vi "Dashboard Main.vi"() -> ()   [LabVIEW 2012]
panel:
  out "Up to Speed":bool
  in  "Tab Control":enum32{"Home", "Debugging"}(tab)
  out "Drive Speed":dbl
  out "Angle of shooter":dbl
  out "Low":bool
  out "Medium":bool
  out "High":bool
  out "Coordinates":cluster{"Y":dbl[], "Y":dbl[]}[](graph)
  out "Speed of shooter":dbl
  out "Distance from target":dbl
  out "Mode":enum8{"Tele-Op", "Auto", "Test", ""}(ring)=enum."Test"
  out "Camera IP":string
  out "JS1 Z":dbl(slide) scale=-1.0..1.0 scale format="%#_2e"
  out "JS2 Z":dbl(slide) scale=-1.0..1.0 scale format="%#_2e"
  out "Joystick 1":cluster{"X":dbl, "Y":dbl}[](graph)
  out "Joystick 2":cluster{"X":dbl, "Y":dbl}[](graph)
  out "JS Buttons 1":T1
  out "JS Buttons 2":T1
  out "MotorSlide4":dbl(slide) scale=-1.0..1.0 scale format="%#_2e"
  out "MotorSlide3":dbl(slide) scale=-1.0..1.0 scale format="%#_2e"
  out "MotorSlide2":dbl(slide) scale=-1.0..1.0 scale format="%#_2e"
  in  "MotorName3":string="Front Left"
  in  "MotorName4":string="Front Right"
  in  "MotorName1":string="Rear Left"
  in  "MotorName2":string="Rear Right"
  out "MotorChart4":dbl(graph)
  out "MotorChart3":dbl(graph)
  out "MotorChart2":dbl(graph)
  out "MotorSlide1":dbl(slide) scale=-1.0..1.0 scale format="%#_2e"
  out "MotorChart1":dbl(graph)
  out "Battery Value":dbl(slide) scale=0.0..14.0 scale format="%#_2e"
  out "Robot IP":string
  out "Battery":sgl(graph)
  in  "Viewer":T2(tab)
  out "Image Error Message":string="Timeout in Camera Communications"
  in  "Video Enable":bool=TRUE
  out "Camera Image":T3(plugin-control)
  out "Buttons 1":cluster{"1":bool, "2":bool, "3":bool}
  out "Kinect 1":cluster{"X":dbl, "Y":dbl, "Z":dbl} {"X" scale=1.0..-1.0; "Y" scale=1.0..-1.0; "Z" scale=1.0..-1.0}
  out "Buttons 2":cluster{"1":bool, "2":bool, "3":bool}
  out "Kinect 2":cluster{"X":dbl, "Y":dbl, "Z":dbl} {"X" scale=1.0..-1.0; "Y" scale=1.0..-1.0; "Z" scale=1.0..-1.0}
  out "Version":string
  out "Skeleton Picture":picture
  out "Players":i8
  out "Tree":string(tree)
  # "Drive & Motors"
  # "Robot IP:"
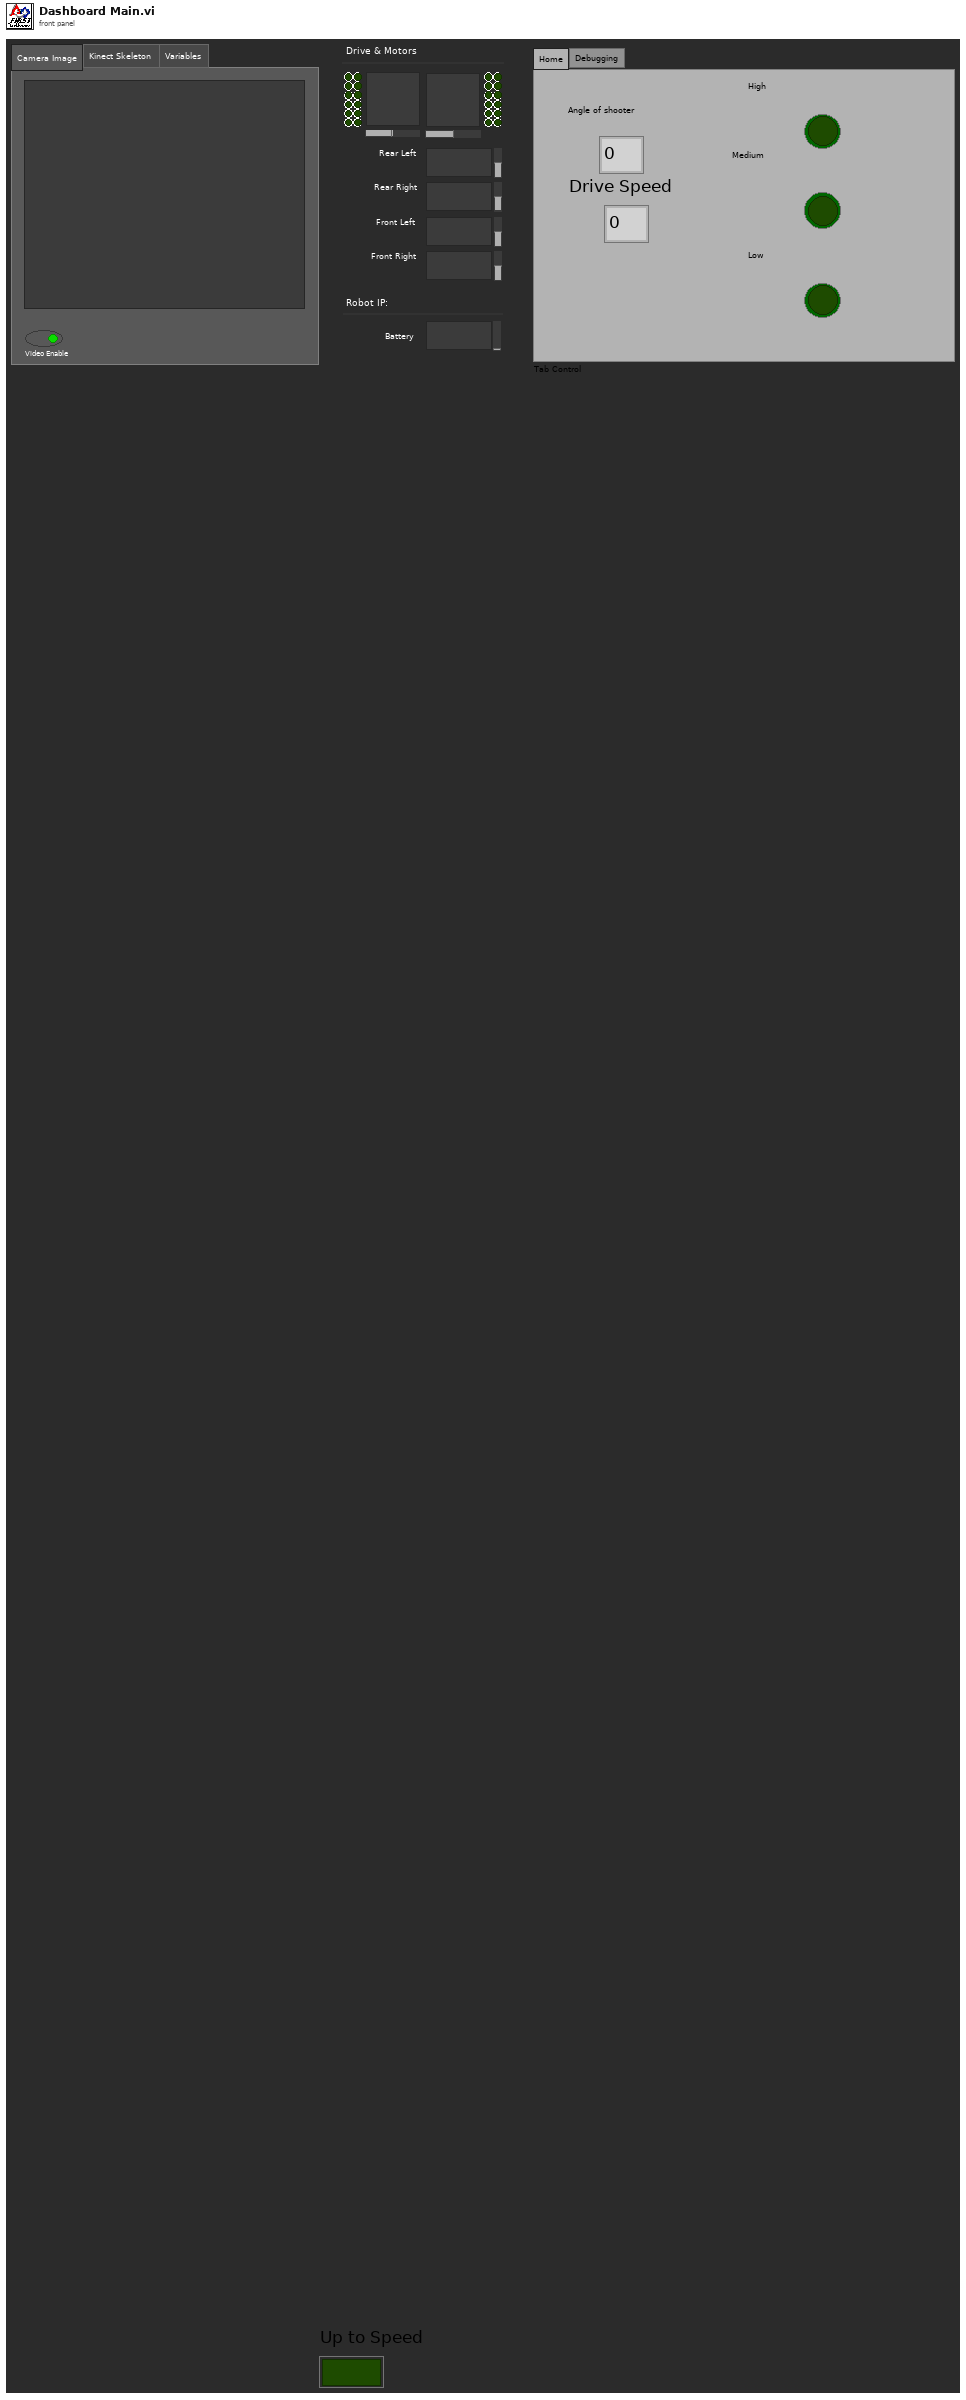
[diagram p1: front panel]
types:
  T1 = cluster{bool, bool, bool, bool, bool, bool, bool, bool, bool, bool, bool, bool}
  T2 = enum32{"Camera Image", "Kinect Skeleton", "Variables"}
  T3 = typedef "IMAQ Image.ctl" = refnum<image>
  T4 = typedef "Image Type" = u32
  T5 = typedef "SkeletonTrackState.ctl" = enum32{"NotTracked", "PositionOnly", "Tracked"}
  T6 = cluster{"TrackingState":u8[], "Position":cluster{"x":sgl, "y":sgl, "z":sgl}, cluster{"x":sgl, "y":sgl, "z":sgl, sgl}[], "TrackState":T5}
  T7 = cluster{cluster{"ScaledToPercentRange":dbl, "ScaledToPercentRange":dbl, "ScaledToPercentRange":dbl}, cluster{bool, bool, bool}}[]
  T8 = typedef "LVBoundsTypeDef.ctl" = cluster{"Width":u32, "Height":u32}
  T9 = cluster{cluster{"ScaledToPercentRange":dbl, "ScaledToPercentRange":dbl, "ScaledToPercentRange":dbl}, cluster{bool, bool, bool}}
  T10 = cluster{"ScaledToPercentRange":dbl, "ScaledToPercentRange":dbl, "ScaledToPercentRange":dbl}
  T11 = typedef "LVRectTypeDef.ctl" = cluster{"Left":i16, "Top":i16, "Right":i16, "Bottom":i16}
  T12 = cluster{"Competition mode":bool, "Robot Link":bool, "Autonomous":bool, "Enabled":bool, "E-Stop":bool, "Simulated":bool, "TestMode":bool, "Docked Window":bool}
  T13 = cluster{"Boolean Array[0]":bool, "Boolean Array[1]":bool, "Boolean Array[2]":bool, "Boolean Array[3]":bool, "Boolean Array[4]":bool, "Boolean Array[5]":bool, "Boolean Array[6]":bool, "Boolean Array[7]":bool, "Boolean Array[8]":bool, "Boolean Array[9]":bool, "Boolean Array[10]":bool, "Boolean Array[11]":bool}
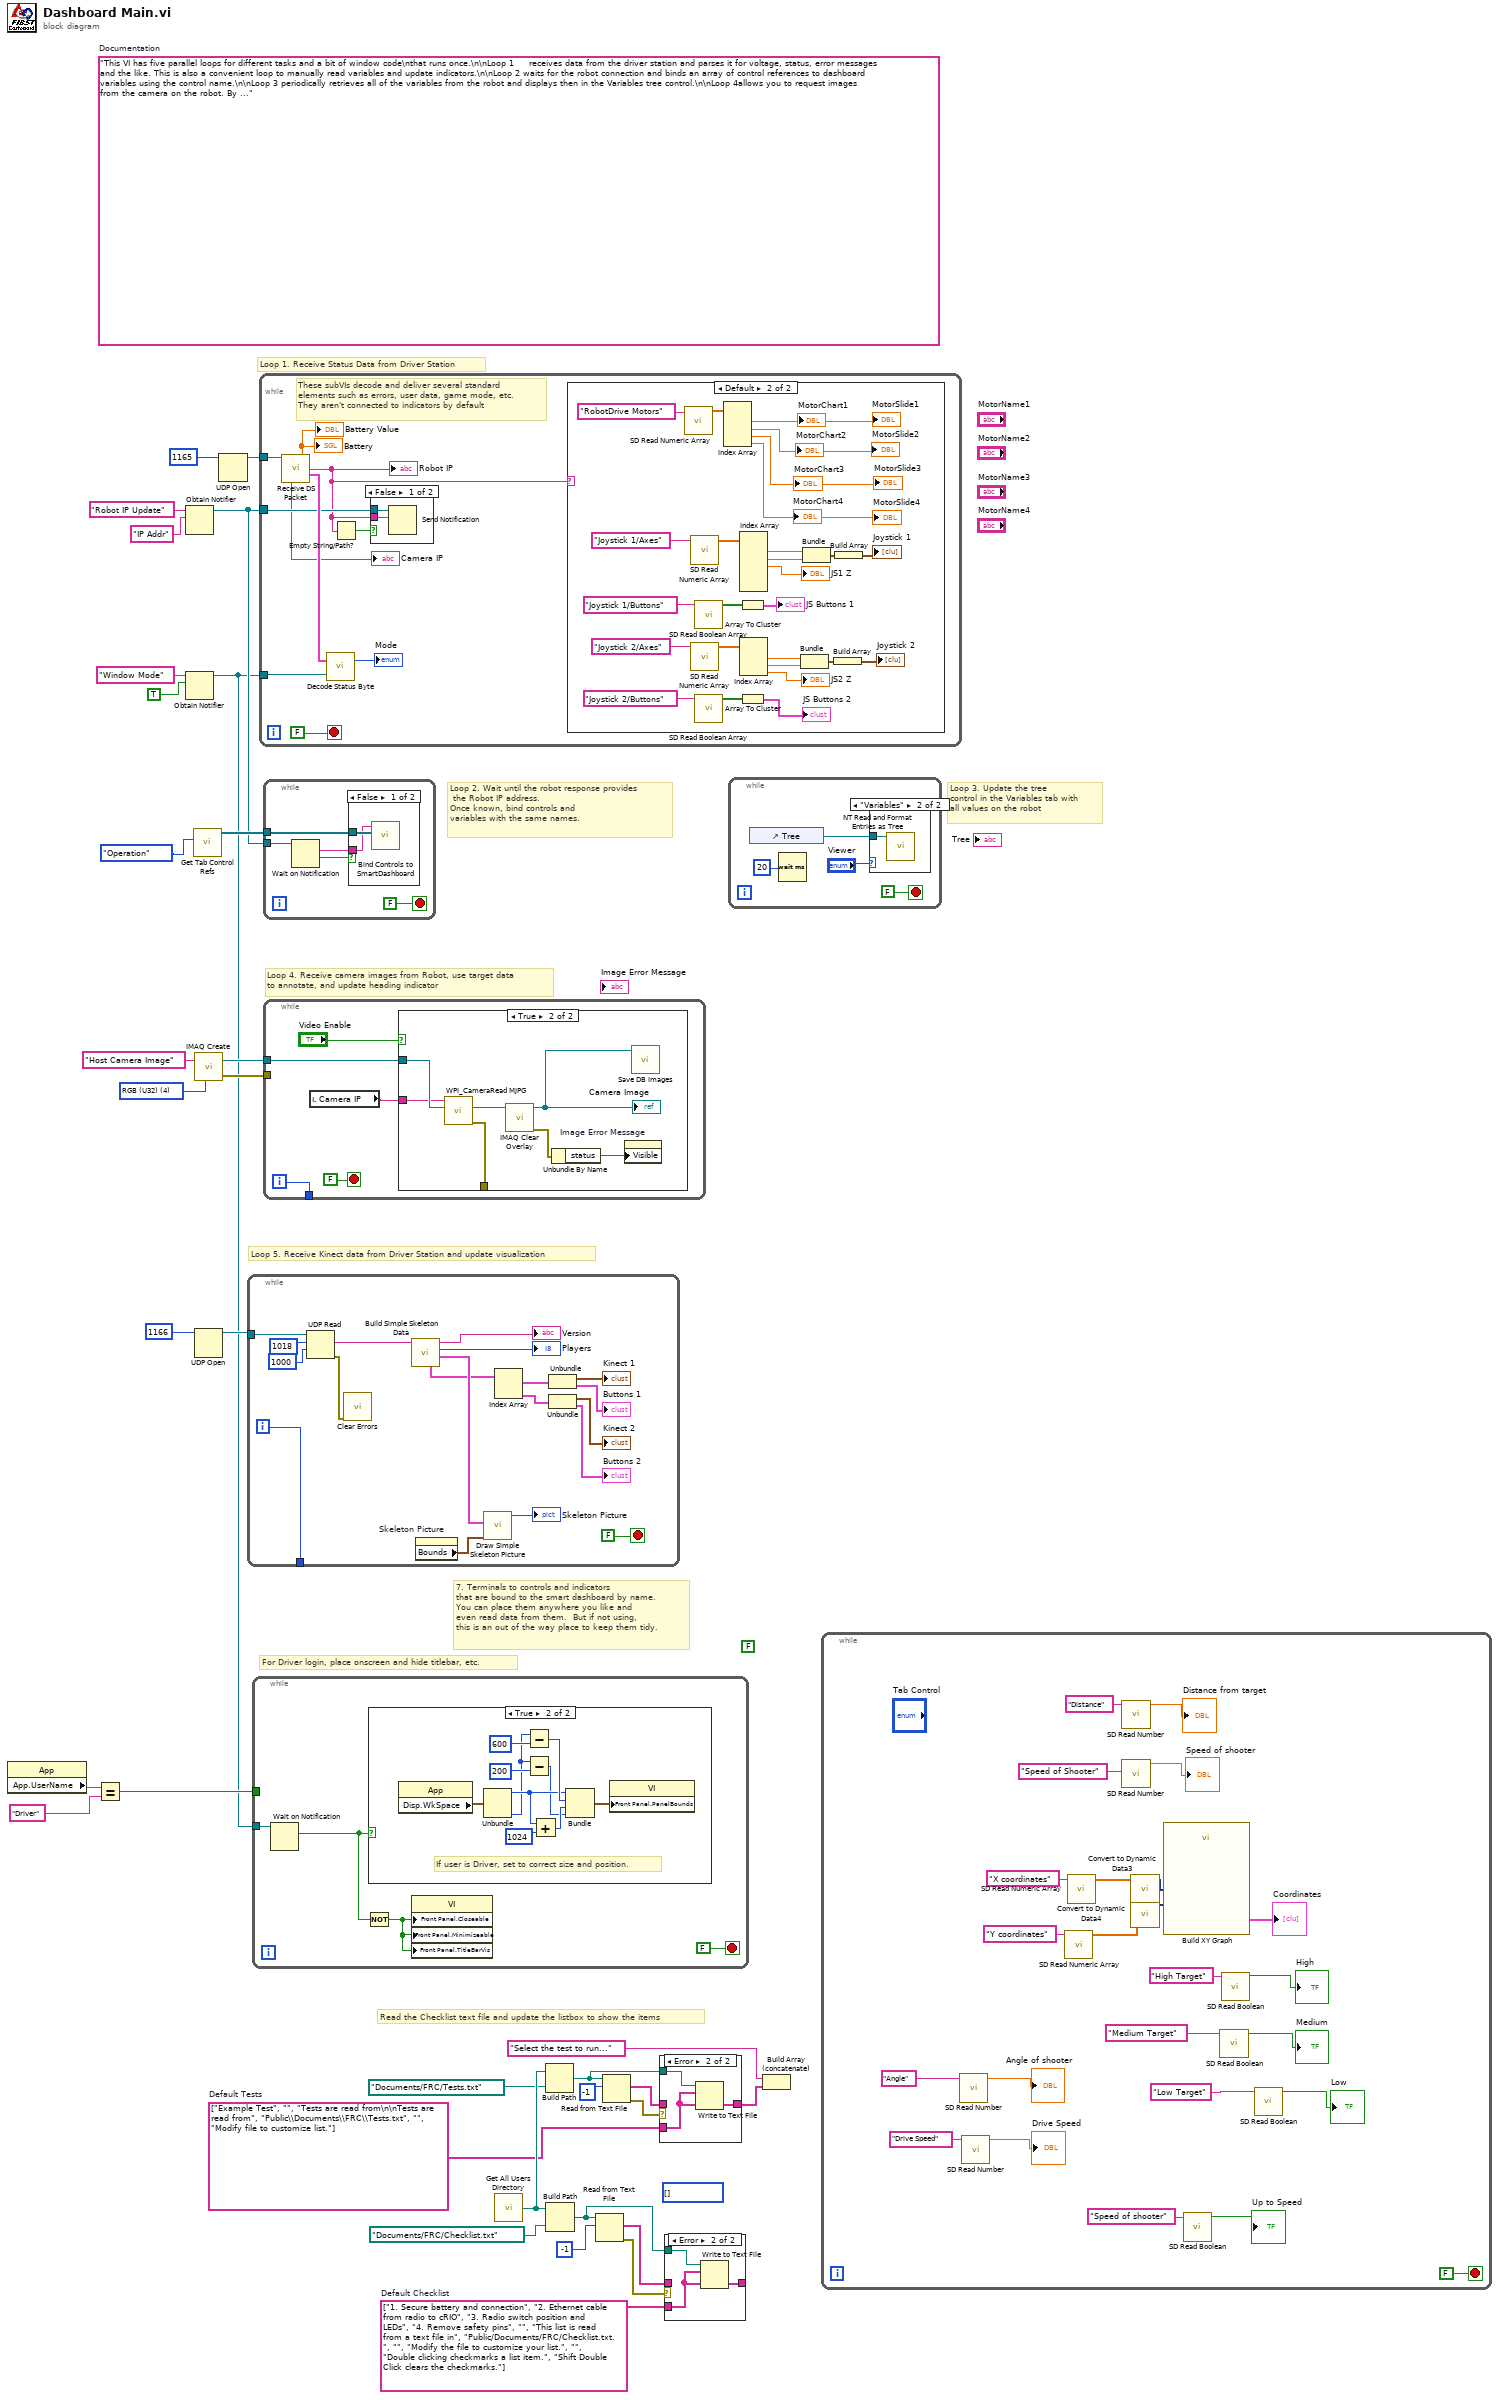
[diagram p0: block diagram]
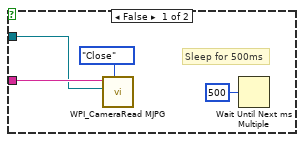
[diagram p9: hidden frame]
diagram:
  w1 = string[] ["1. Secure battery and connection", "2. Ethernet cable from radio to cRIO", "3. Radio switch position and LEDs", "4. Remove safety pins", "", "This list is read from a text file in", "Public/Documents/FRC/Checklist.txt.", "", "Modify the file to customize your list.", "", "Double clicking checkmarks a list item.", "Shift Double Click clears the checkmarks."]  # Default Checklist
  w6 = string[] ["Example Test", "", "Tests are read from\n\nTests are read from", "Public\\Documents\\FRC\\Tests.txt", "", "Modify file to customize list."]  # Default Tests
  (unwired) FALSE ("Visible")
  (unwired) i32[] [] ("Item Symbols")
  (unwired) "This VI has five parallel loops for different tasks and a bit of window code\nthat runs once.\n\nLoop 1     receives data from the driver station and parses it for voltage, status, error messages and the like. This is also a convenient loop to manually read variables and update indicators.\n\nLoop 2 waits for the robot connection and binds an array of control references to dashboard variables using the control name.\n\nLoop 3 periodically retrieves all of the variables from the robot and displays then in the Variables tree control.\n\nLoop 4allows you to request images from the camera on the robot. By default, it reads the images using MJPG stream, but has compatibility for the older setup which used JPGs.\n\nLoop 5 processes any data from the Kinect server and shows the skeleton and Kinect stick values in the Kinect tab.\n\nLoop 6 process events for the TestMode tree, listbox, ring, and actuator\n\nLoop 7 calculates and updates the window location, size, and style. The checklist and tests are loaded from text files and placed into the controls.\n\nAdding new indicators or controls:\nAdd them to the panel in the Operations tab and name them the same as the SmartDashboard variable on the robot. The binding loop will keep them synchronized."  # Documentation
  w32 = T4 4 items=["Grayscale (U8)", "Grayscale (I16)", "Grayscale (SGL)", "Complex (CSG)", "RGB (U32)", "HSL (U32)", "RGB (U64)"] ("Image Type")
  # "Read the Checklist text file and update the listbox to show the items"
  # "7. Terminals to controls and indicators\nthat are bound to the smart dashboard by name.\nYou can place them anywhere you like and\neven read data from them.  But if not using,\nthis is an out of the way place to keep them tidy."
  # "Loop 3. Update the tree\ncontrol in the Variables tab with\nall values on the robot"
  # "Loop 2. Wait until the robot response provides\n the Robot IP address.\nOnce known, bind controls and\nvariables with the same names."
  # "Loop 5. Receive Kinect data from Driver Station and update visualization"
  # "For Driver login, place onscreen and hide titlebar, etc."
  # "Loop 1. Receive Status Data from Driver Station"
  # "Loop 4. Receive camera images from Robot, use target data\nto annotate, and update heading indicator"
  n1 = property class="App"() -> ("App.UserName"=w27:string)  [unwired: 2 in, 2 out]
  n2 = Equal?(x=w27, y="Driver") -> (x = y?=w26:bool)
  n3 = Obtain Notifier(name (unnamed)="Robot IP Update", notification data type="IP Addr" ("name (unnamed)")) -> (notifier out=w20:refnum<notifier>)  [unwired: 2 in, 2 out]
  n4 = Obtain Notifier(name (unnamed)="Window Mode", notification data type=TRUE) -> (notifier out=w10:refnum<notifier>)  [unwired: 2 in, 2 out]
  n5 = call <vilib>:"Get Tab Control Refs.vi"("Page Index"=enum32{"Operation", "Test"}."Operation" ("Dashboard Tab")) -> ("ControlsOnPage"=w23:refnum<vi>[])  [unwired: 10 in]
  n6 = call "IMAQ Create"("Image Name"="Host Camera Image", "Image Type"=w32) -> ("New Image"=w30:T3, "error out"=w29:errorcluster)  [unwired: 2 in, 1 out]
  n7 = UDP Open(11:u16 1166 ("port")) -> (port=w24:refnum<k16>)  [unwired: 2 in, 4 out]
  n8 = UDP Open(11:u16 1165 ("port")) -> (port=w33:refnum<k16>)  [unwired: 2 in, 4 out]
  n9 = while {
    tunnel: w24 -> [w51]
    tunnel: [w35] -> _
    i -> [w35]
    stop <- FALSE stop-if-true
    n10 = UDP Read(connection ID=w51, max size (548)=1018 ("bytes to read"), timeout ms (25000)=1000) -> (data out=w45:string, error out=w43:errorcluster)  [unwired: 1 in, 3 out]
    n11 = call <vilib>:"Clear Errors.vi"("error in (no error)"=w43) -> ()  [unwired: 6 in, 1 out]
    n12 = call "Build Simple Skeleton Data.vi"("data out"=w45) -> ("Skeleton Data"=w46:T6, "NumPlayers"=→"Players":i8, "Version String"=→"Version":string, "Simple Joystick Info"=w42:T7)  [unwired: 6 in, 1 out]
    n13 = property on="Skeleton Picture" class="Pict"() -> ("Bounds"=w47:T8)  [unwired: 2 in, 2 out]
    n14 = call "Draw Simple Skeleton Picture.vi"("Bounds"=w47, "Simple Skeleton"=w46) -> ("new picture out"=→"Skeleton Picture":picture)  [unwired: 9 in]
    n15 = Index Array(array=w42) -> (element #1=w41:T9, element #2=w40:T9)  [unwired: 2 in]
    n16 = Unbundle(w41) -> (→"Kinect 1":T10, →"Buttons 1":cluster{bool, bool, bool})
    n17 = Unbundle(w40) -> (→"Kinect 2":T10, →"Buttons 2":cluster{bool, bool, bool})
  }
  n18 = while {
    tunnel: w26 -> [_]
    tunnel: w10 -> [w56]
    stop <- FALSE stop-if-true
    n19 = Wait on Notification(notifier=w56) -> (notification=w54:bool)  [unwired: 3 in, 3 out]
    n20 = Not(x=w54) -> (.not. x?=w55:bool)
    n21 = case shown="True" w54 {
      frame False {
      }
      frame True {
        # "If user is Driver, set to correct size and position."
        n22 = property class="App"() -> ("Disp.WkSpace"=w67:T11)  [unwired: 2 in, 2 out]
        n23 = Unbundle(w67) -> ("Left"=w62:i16, "Bottom"=w58:i16)  [unwired: 2 out]
        n24 = Subtract(x=w58, y=600) -> (x-y=w64:i32)
        n25 = Subtract(x=w58, y=200) -> (x-y=w59:i32)
        n26 = Add(x=w62, y=1024) -> (x+y=w63:i32)
        n27 = Bundle("Left"=w62, w64, w63, w59) -> (w66:cluster{"Left":i16, i32, i32, i32})  [unwired: 1 out]
        n28 = property class="VI"("Front Panel.PanelBounds"=w66) -> ()  [unwired: 2 in, 2 out]
      }
    }
    n29 = property class="VI"("Front Panel.Closeable"=w55, "Front Panel.Minimizeable"=w55, "Front Panel.TitleBarVis"=w55) -> ()  [unwired: 2 in, 2 out]
  }
  n30 = while {
    tunnel: w33 -> [w75]
    tunnel: w20 -> [w73]
    tunnel: w10 -> [w70]
    stop <- FALSE stop-if-true
    # "These subVIs decode and deliver several standard\nelements such as errors, user data, game mode, etc.\nThey aren't connected to indicators by default"
    n31 = call "Receive DS Packet.vi"("Recv Socket"=w75) -> ("Battery"=→"Battery" →"Battery Value":sgl, "Robot IP Address"=w72:string, "Status"=w76:T12, "Camera IP Address"=→"Camera IP":string)  [unwired: 1 in, 10 out]
    "Robot IP" <- w72
    n32 = call "Decode Status Byte.vi"("Window Mode Notifier"=w70, "Status"=w76) -> ("Mode"=→"Mode":enum8{"Tele-Op", "Auto", "Test", ""})  [unwired: 1 out]
    n33 = Empty String/Path?(string/path=w72) -> (empty?=w71:bool)
    n34 = case shown="False" w71 {
      tunnel: w73 -> [w105 _]
      tunnel: w72 -> [w104 _]
      frame False {
        n35 = Send Notification(notification=w104, notifier=w105) -> ()  [unwired: 1 in, 2 out]
      }
      frame True {
      }
    }
    n36 = case shown="Default" w72 {
      frame "" {
        # "Robot not responding, don't poll the variables"
      }
      frame Default {
        n37 = call <vilib>:"SD Read Numeric Array.vi"("Name"="RobotDrive Motors") -> ("Numeric Array"=w100:dbl[])  [unwired: 8 in, 2 out]
        n38 = call <vilib>:"SD Read Numeric Array.vi"("Name"="Joystick 1/Axes") -> ("Numeric Array"=w93:dbl[])  [unwired: 8 in, 2 out]
        n39 = call <vilib>:"SD Read Numeric Array.vi"("Name"="Joystick 2/Axes") -> ("Numeric Array"=w87:dbl[])  [unwired: 8 in, 2 out]
        n40 = call <vilib>:"SD Read Boolean Array.vi"("Name"="Joystick 1/Buttons") -> ("Boolean Array"=w95:bool[])  [unwired: 8 in, 2 out]
        n41 = call <vilib>:"SD Read Boolean Array.vi"("Name"="Joystick 2/Buttons") -> ("Boolean Array"=w86:bool[])  [unwired: 8 in, 2 out]
        n42 = Index Array(array=w100) -> (element #1=→"MotorChart1" →"MotorSlide1":dbl, element #2=→"MotorSlide2" →"MotorChart2":dbl, element #3=→"MotorChart3" →"MotorSlide3":dbl, element #4=→"MotorChart4" →"MotorSlide4":dbl)  [unwired: 4 in]
        n43 = Array To Cluster(array=w95) -> (cluster=→"JS Buttons 1":T13)
        n44 = Array To Cluster(array=w86) -> (cluster=→"JS Buttons 2":T13)
        n45 = Index Array(array=w93) -> (element #1=w90:dbl, element #2=w91:dbl, element #3=→"JS1 Z":dbl)  [unwired: 6 in, 3 out]
        n46 = Index Array(array=w87) -> (element #1=w82:dbl, element #2=w81:dbl, element #3=→"JS2 Z":dbl)  [unwired: 3 in]
        n47 = Bundle("Numeric"=w82, "Numeric"=w81) -> (w83:cluster{"Numeric":dbl, "Numeric":dbl})  [unwired: 1 in]
        n48 = Bundle("Numeric"=w90, "Numeric"=w91) -> (w89:cluster{"Numeric":dbl, "Numeric":dbl})  [unwired: 1 in]
        n49 = Build Array(w83) -> (→"Joystick 2":cluster{"Numeric":dbl, "Numeric":dbl}[])
        n50 = Build Array(w89) -> (→"Joystick 1":cluster{"Numeric":dbl, "Numeric":dbl}[])
      }
    }
  }
  n51 = while {
    tunnel: w23 -> [w110]
    tunnel: w20 -> [w107]
    stop <- FALSE stop-if-true
    n52 = Wait on Notification(notifier=w107) -> (notification=w106:string, timed out?=w108:bool)  [unwired: 3 in, 2 out]
    n53 = case shown="False" w108 {
      tunnel: w110 -> [w112 _]
      tunnel: w106 -> [w111 _]
      frame False {
        n54 = call <vilib>:"Bind Controls to SmartDashboard.vi"("Bound Control Refs"=w112, "Server IP Address"=w111) -> ()  [unwired: 10 in]
      }
      frame True {
      }
    }
  }
  n55 = while {
    tunnel: w30 -> [w116]
    tunnel: w29 -> [_]
    tunnel: [w114] -> _
    i -> [w114]
    stop <- FALSE stop-if-true
    n56 = local read "Camera IP"() -> (w113:string)
    n57 = case shown="True" "Video Enable" {
      tunnel: w113 -> [w120 w122]
      tunnel: w116 -> [w119 w128]
      tunnel: [_ w123] -> _
      frame False {
        # "Sleep for 500ms"
        n58 = call <vilib>:"WPI_CameraRead MJPG.vi"("Operation"=enum16{"Read", "Reopen", "Close"}."Close", "Image"=w119, "address"=w120) -> ()  [unwired: 7 in, 2 out]
        n59 = Wait Until Next ms Multiple(millisecond multiple=u32 500) -> ()  [unwired: 1 out]
      }
      frame True {
        n60 = call <vilib>:"WPI_CameraRead MJPG.vi"("Image"=w128, "address"=w122) -> ("error out"=w123:errorcluster, "Image Out"=w125:T3)  [unwired: 8 in]
        n61 = call "IMAQ Clear Overlay"("Image"=w125) -> ("error out"=w126:errorcluster, "Image Out"=w124:T3)  [unwired: 2 in, 7 out]
        "Camera Image" <- w124
        n62 = Unbundle By Name(w126) -> ("status"=w127:bool)
        n63 = property on="Image Error Message" class="Str"("Visible"=w127) -> ()  [unwired: 2 in, 2 out]
        n64 = call "Save DB Images.vi"("Image"=w124) -> ()  [unwired: 2 in, 1 out]
      }
    }
  }
  n65 = call "Get All Users Directory.vi"() -> ("All User Path"=w16:path)
  n66 = Build Path(base path=w16, name or relative path=path "Documents/FRC/Tests.txt") -> (appended path=w5:path)
  n67 = Build Path(base path=w16, name or relative path=path "Documents/FRC/Checklist.txt") -> (appended path=w2:path)
  n68 = Read from Text File(file (use dialog)=w2, count=-1 ("timeout ms (25000)")) -> (text=w3:string[], error out=w4:errorcluster)  [unwired: 2 in, 2 out]
  n69 = Read from Text File(file (use dialog)=w5, count=-1 ("timeout ms (25000)")) -> (text=w8:string[], error out=w9:errorcluster)  [unwired: 2 in, 2 out]
  n70 = case shown="Error" w9 {
    tunnel: w8 -> [w129 _]
    tunnel: [w129 w130] -> w7
    tunnel: w6 -> [_ w130]
    tunnel: w5 -> [_ w131]
    frame No Error {
    }
    frame Error {
      n71 = Write to Text File(file (use dialog)=w131, text=w130) -> ()  [unwired: 2 in, 3 out]
    }
  }
  n72 = case shown="Error" w4 {
    tunnel: w3 -> [w132 _]
    tunnel: [w132 w133] -> _
    tunnel: w1 -> [_ w133]
    tunnel: w2 -> [_ w134]
    frame No Error {
    }
    frame Error {
      n73 = Write to Text File(file (use dialog)=w134, text=w133) -> ()  [unwired: 2 in, 3 out]
    }
  }
  n74 = while {
    stop <- FALSE stop-if-true
    n75 = control-ref of="Tree"() -> (w136:refnum<vi>)
    n76 = Wait (ms)(milliseconds to wait=u32 20) -> ()  [unwired: 1 out]
    n77 = case shown="\"Variables\"" "Viewer" {
      tunnel: w136 -> [_ w139]
      frame "Camera Image", Default {
      }
      frame "Variables" {
        n78 = call <vilib>:"NT Read and Format Entries as Tree.vi"("Tree Refnum"=w139) -> ()  [unwired: 9 in, 2 out]
      }
    }
  }
  n79 = Build Array (concatenate)("Select the test to run...", w7) -> ()  [unwired: 1 out]
  n80 = while {
    stop <- FALSE stop-if-true
    n81 = call <vilib>:"SD Read Number.vi"("Name"="Angle") -> ("Numeric"=→"Angle of shooter":dbl)  [unwired: 8 in, 2 out]
    n82 = call <vilib>:"SD Read Number.vi"("Name"="Drive Speed") -> ("Numeric"=→"Drive Speed":dbl)  [unwired: 8 in, 2 out]
    n83 = call <vilib>:"SD Read Numeric Array.vi"("Name"="Y coordinates") -> ("Numeric Array"=w158:dbl[])  [unwired: 8 in, 2 out]
    n84 = call <vilib>:"SD Read Numeric Array.vi"("Name"="X coordinates") -> ("Numeric Array"=w160:dbl[])  [unwired: 8 in, 2 out]
    n85 = call <vilib>:"SD Read Number.vi"("Name"="Distance") -> ("Numeric"=→"Distance from target":dbl)  [unwired: 8 in, 2 out]
    n86 = call <vilib>:"SD Read Number.vi"("Name"="Speed of Shooter") -> ("Numeric"=→"Speed of shooter":dbl)  [unwired: 8 in, 2 out]
    n87 = call "Convert to Dynamic Data3"("Array"=w160) -> ("Dynamic Data Type"=w159:dynamicdata)  [unwired: 3 in]
    n88 = call "Convert to Dynamic Data4"("Array"=w158) -> ("Dynamic Data Type"=w157:dynamicdata)  [unwired: 3 in]
    n89 = call "Build XY Graph"("Y Input"=w157, "X Input"=w159) -> ("XY Graph"=→"Coordinates":cluster{"Y":dbl[], "Y":dbl[]}[])  [unwired: 3 in, 6 out]
    n90 = call <vilib>:"SD Read Boolean.vi"("Name"="Speed of shooter") -> ("Boolean"=→"Up to Speed":bool)  [unwired: 8 in, 2 out]
    n91 = call <vilib>:"SD Read Boolean.vi"("Name"="Medium Target") -> ("Boolean"=→"Medium":bool)  [unwired: 8 in, 2 out]
    n92 = call <vilib>:"SD Read Boolean.vi"("Name"="High Target") -> ("Boolean"=→"High":bool)  [unwired: 8 in, 2 out]
    n93 = call <vilib>:"SD Read Boolean.vi"("Name"="Low Target") -> ("Boolean"=→"Low":bool)  [unwired: 8 in, 2 out]
  }
